vi "Stop.vi"(8 "error in (no error)":errorcluster, 11 "DVR in":refnum<class "Data Server.lvclass">) -> (0 "error out":errorcluster)   [LabVIEW 2020, in "Veristandgrpc_server.lvlib" / "Data Server.lvclass"]
uses:
  Data Server.lvclass
  Data Server.lvclass/Data Server.ctl
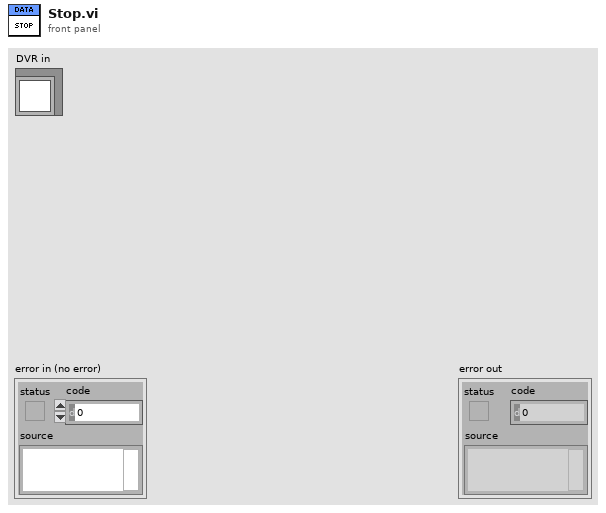
[diagram p1: front panel]
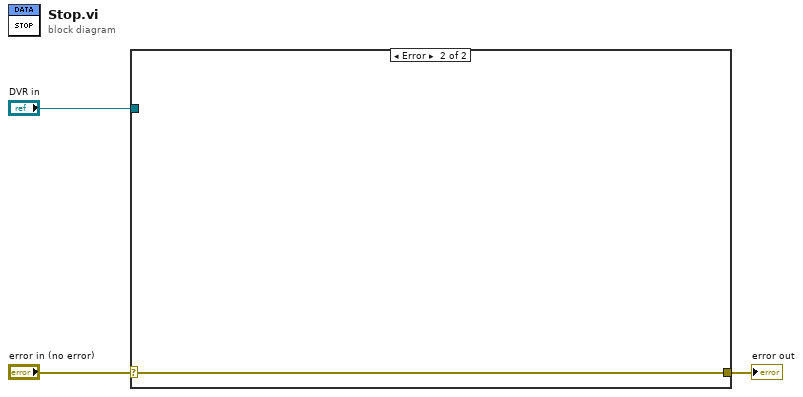
[diagram p0: block diagram]
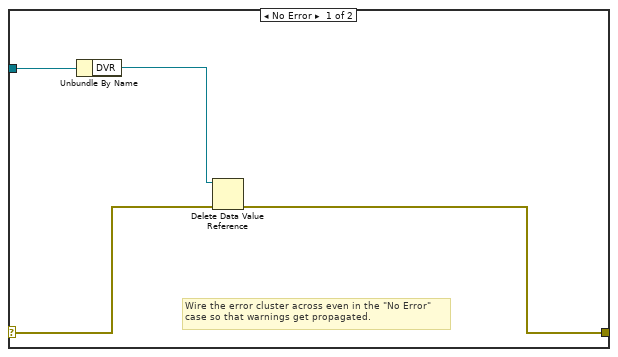
[diagram p2: hidden frame]
diagram:
  n1 = case shown="Error" "error in (no error)" {
    selector: "error in (no error)" -> [w5 w8]
    tunnel: [w4 w8] -> w2
    tunnel: "DVR in" -> [w7 _]
    frame No Error {
      # "Wire the error cluster across even in the \"No Error\"\ncase so that warnings get propagated."
      n2 = Unbundle By Name(w7) -> ("DVR"=w6:refnum<data-value>)
      n3 = Delete Data Value Reference(data value reference=w6, error in=w5) -> (error out=w4:errorcluster)  [unwired: 1 out]
    }
    frame Error {
    }
  }
  "error out" <- w2
